vi "new write.vi"(8 "Next Floor":string="Ground Floor: ", 9 "Current Floor":T1, 10 "Counter Value in":i32, 11 "Byte Stream File in":refnum<file>) -> (0 "error out":errorcluster, 2 "Written String":string)   [LabVIEW 2017]
uses:
  Working Demo Phase/Current Floor.ctl
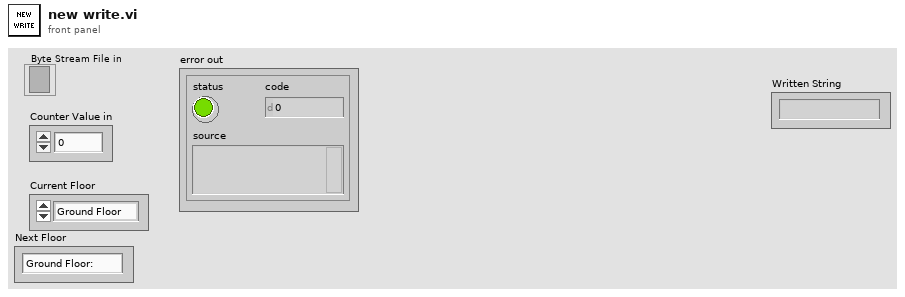
[diagram p1: front panel]
types:
  T1 = typedef "Current Floor.ctl" = enum16{"Ground Floor", "Floor 1", "Floor 2"}
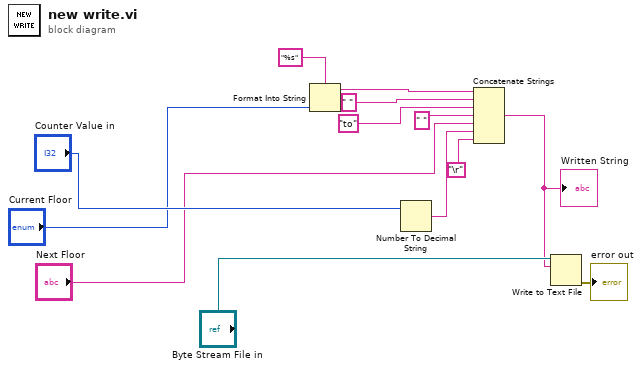
[diagram p0: block diagram]
diagram:
  n1 = Format Into String(format string="%s", "Current Floor") -> (resulting string=w4:string)  [unwired: 2 in, 1 out]
  n2 = Number To Decimal String(number="Counter Value in") -> (decimal integer string=w9:string)  [unwired: 1 in]
  n3 = Concatenate Strings(w4, " " ("string"), "to" ("string"), " " ("string"), "Next Floor", w9, "\r") -> (w6:string)
  "Written String" <- w6
  n4 = Write to Text File(file (use dialog)="Byte Stream File in", text=w6) -> (error out=→"error out":errorcluster)  [unwired: 2 in, 2 out]
